vi "Read Configuration Class Name.vi"(8 "error in":errorcluster, 11 "TEC editor node in":refnum<class "TEC editor node.lvclass">) -> (0 "error out":errorcluster, 2 "Class Name":string, 3 "TEC editor node out":refnum<class "TEC editor node.lvclass">)   [LabVIEW 2013, in "TEC editor node.lvclass"]
uses:
  TEC editor node.lvclass
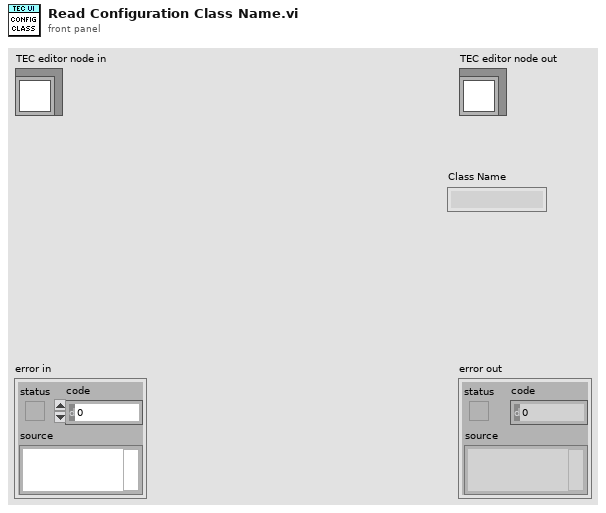
[diagram p1: front panel]
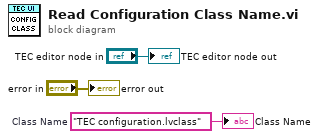
[diagram p0: block diagram]
diagram:
  w1 = "TEC configuration.lvclass"  # Class Name
  "error out" <- "error in"
  "TEC editor node out" <- "TEC editor node in"
  "Class Name" <- w1
